vi "脉冲测量_基于滴答__连续.vi"() -> ()   [LabVIEW 2013]
uses:
  <userlib>/ArtDAQ/_SubVI/ArtDAQ_CreateCIPulseChanTicks.vi
  <userlib>/ArtDAQ/_SubVI/ArtDAQ_CfgImplicitTiming.vi
  <userlib>/ArtDAQ/_SubVI/ArtDAQ_Read Counter Tick NSamp.vi
panel:
  in  "时钟滴答源":string="100MHzTimebase"
  out "低滴答数":u32[](array[numeric])
  in  "每通道点数":i32=1000
  in  "停止":bool
  out "高滴答数":u32[](array[numeric])
  in  "计数器":string="Dev1/ctr0"
  in  "最小值":dbl=2.0 format="%0.6f"
  in  "最大值":dbl=2000000.0 format="%0.6f"
  out "错误输出":errorcluster
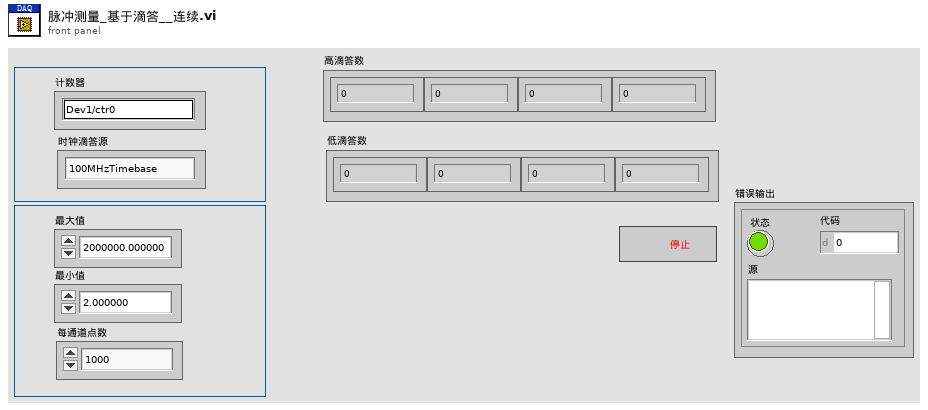
[diagram p1: front panel]
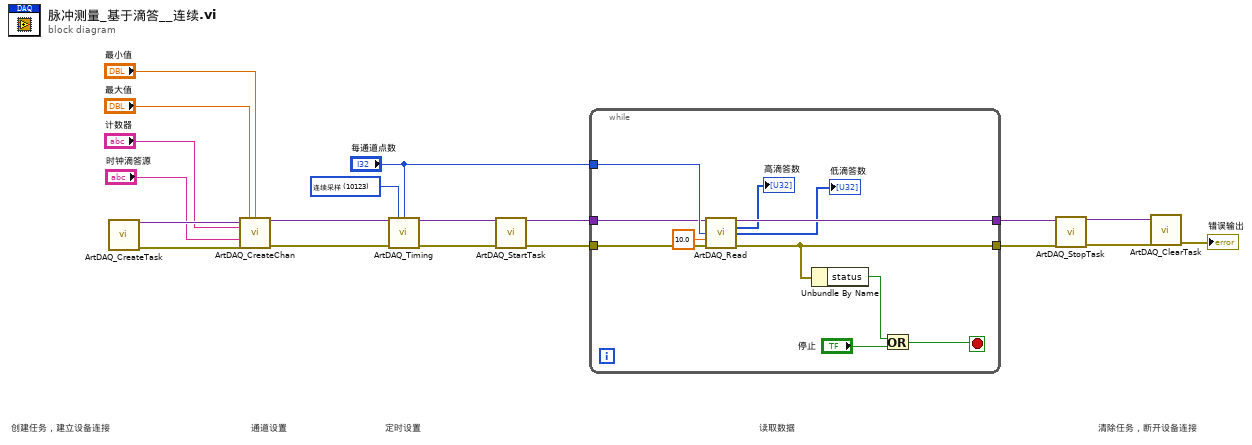
[diagram p0: block diagram]
diagram:
  w7 = 10123 items=["有限点采样"=10178, "连续采样"=10123] ("SampleMode")
  # "通道设置"
  # "创建任务，建立设备连接"
  # "定时设置"
  # "读取数据"
  # "清除任务，断开设备连接"
  n1 = call <userlib>:"ArtDAQ_CreateTask.vi"() -> ("任务句柄"=w19:variant, "错误输出"=w18:errorcluster)  [unwired: 14 in]
  n2 = call-poly <userlib>:"ArtDAQ_CreateChan.vi"("任务句柄"=w19, "最大值"="最大值", "最小值"="最小值", "计数器"="计数器", "时钟滴答源"="时钟滴答源", "错误输入"=w18) -> ("任务句柄"=w9:variant, "错误输出"=w8:errorcluster)  [unwired: 8 in]
  n3 = call-poly <userlib>:"ArtDAQ_Timing.vi"("任务句柄"=w9, "采样模式"=w7, "每通道采样数"="每通道点数", "错误输入"=w8) -> ("任务句柄"=w5:variant, "错误输出"=w4:errorcluster)  [unwired: 10 in]
  n4 = call <userlib>:"ArtDAQ_StartTask.vi"("任务句柄"=w5, "错误输入"=w4) -> ("任务句柄"=w3:variant, "错误输出"=w2:errorcluster)  [unwired: 12 in]
  n5 = while {
    tunnel: [w30] -> w16
    tunnel: [w29] -> w14
    tunnel: "每通道点数" -> [w28]
    tunnel: w3 -> [w23]
    tunnel: w2 -> [w22]
    stop <- w21 stop-if-true
    n6 = call-poly <userlib>:"ArtDAQ_Read.vi"("任务句柄"=w23, "每通道采样数"=w28, "超时s"=10.0 ("Timeout"), "错误输入"=w22) -> ("任务句柄"=w30:variant, "高时钟滴答"=→"高滴答数":u32[], "低时钟滴答"=→"低滴答数":u32[], "错误输出"=w29:errorcluster)  [unwired: 8 in]
    n7 = Unbundle By Name(w29) -> ("status"=w25:bool)
    n8 = Or(x=w25, y="停止") -> (x .or. y?=w21:bool)
  }
  n9 = call <userlib>:"ArtDAQ_StopTask.vi"("任务句柄"=w16, "错误输入"=w14) -> ("任务句柄"=w15:variant, "错误输出"=w13:errorcluster)  [unwired: 12 in]
  n10 = call <userlib>:"ArtDAQ_ClearTask.vi"("任务句柄"=w15, "错误输入"=w13) -> ("错误输出"=→"错误输出":errorcluster)  [unwired: 13 in]
